vi "Actor Core.vi"(8 "error in":errorcluster, 11 "Display in":refnum<class "Display.lvclass">) -> (0 "error out":errorcluster, 3 "Actor out":refnum<class "Actor.lvclass">)   [LabVIEW 2015, in "UserManagement.lvlib" / "Display.lvclass"]
doc: "(<B>Filename</B>: Actor Framework.lvlib:Actor.lvclass:Actor Core.vi)\n\nReceives messages to the actor, reacts to them, and initiates any error handling that may shut the actor down.\n\nDescendant classes may override this VI to append parallel tasks for the actor to complete while it handles messages. Overrides use the Call Parent Method node."
uses:
  Display.lvclass
  <vilib>/ActorFramework/Actor/Actor.lvclass
  typedef/Main Ctl and UI Ref.ctl
  DatabaseManagement/Database.lvclass
  Display.lvclass/Display.ctl
  userInfoManage/UserInfoManageUI.lvclass
  <vilib>/ActorFramework/Actor/Actor.lvclass/Actor.ctl
  <vilib>/ActorFramework/Message Enqueuer/Message Enqueuer.lvclass/Message Enqueuer.ctl
  Messages/Launch Plugin_Msg/Launch Plugin_Msg.lvclass/Launch Plugin_Msg.ctl
  <vilib>/ActorFramework/Message Enqueuer/Init from Existing Queue.vi
  <vilib>/ActorFramework/Message Enqueuer/Enqueue.vi
  <vilib>/ActorFramework/Message Priority Queue/Priority Enqueue.vi
  <vilib>/ActorFramework/Message Enqueuer/Message Enqueuer.lvclass
  Messages/Launch Plugin_Msg/Launch Plugin_Msg.lvclass
panel:
  out "Info":string
  in  "Tab Control":enum32{"CommonUser", "Admin"}(tab)
  in  "WatchPersonRecord":bool
  in  "Request":bool
  in  "ManageInfo":bool
  in  "WatchEntailInfo":bool
  in  "MakePrintTable":bool
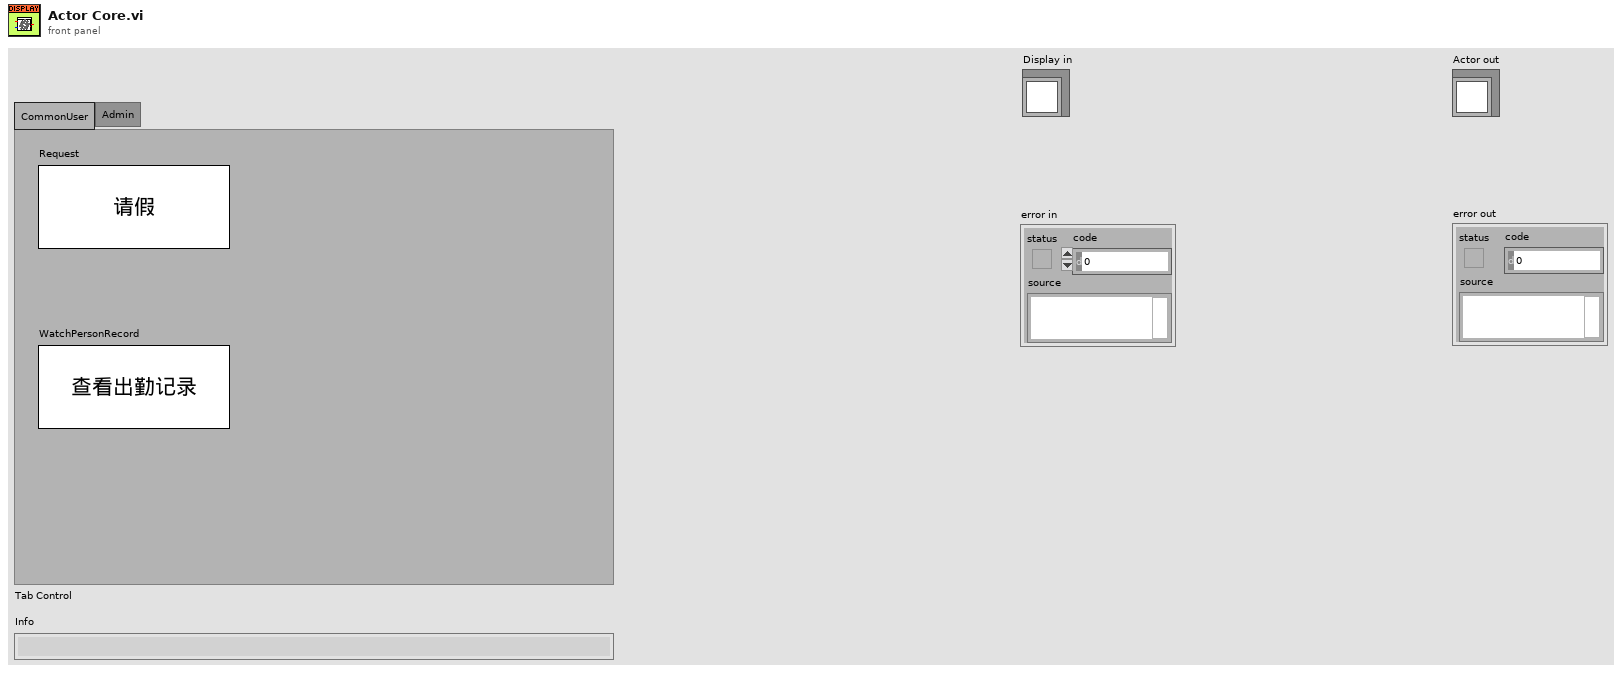
[diagram p1: front panel]
types:
  T1 = typedef "Main Ctl and UI Ref.ctl" = cluster{"Tab Control":refnum<vi>, "Info":refnum<vi>, "This VI":refnum<vi>}
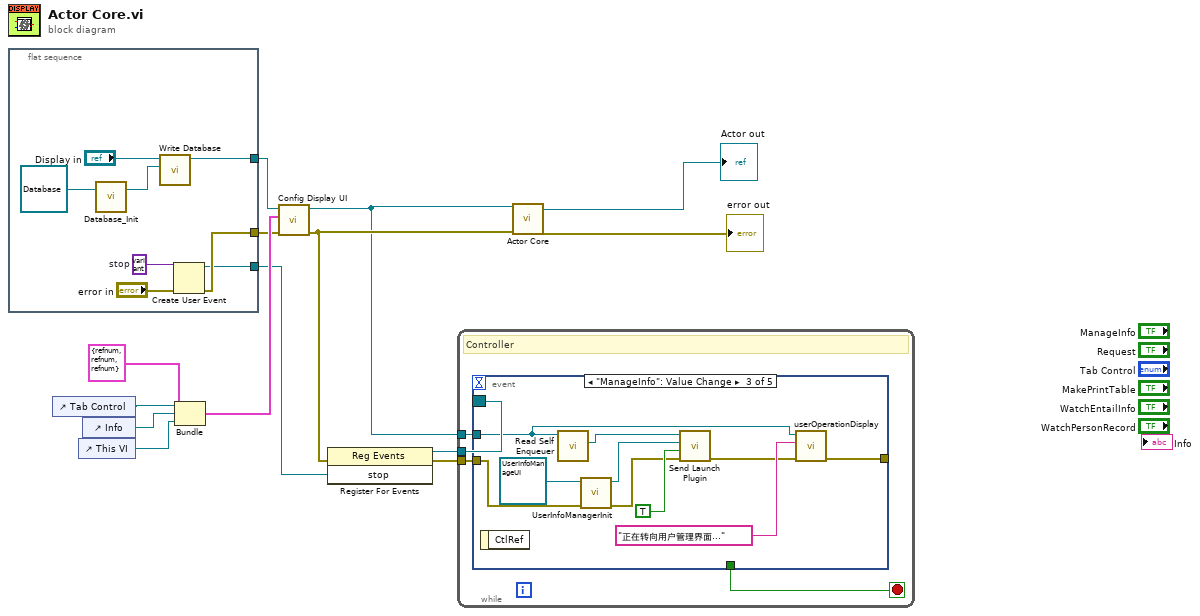
[diagram p0: block diagram]
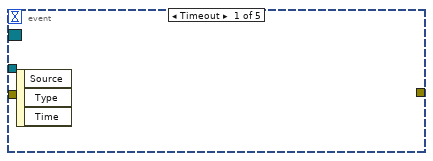
[diagram p2: hidden frame]
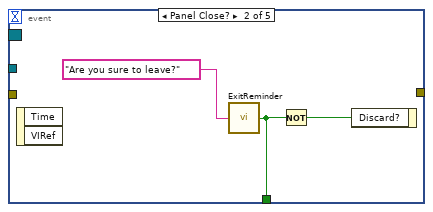
[diagram p3: hidden frame]
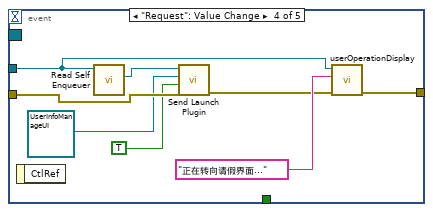
[diagram p4: hidden frame]
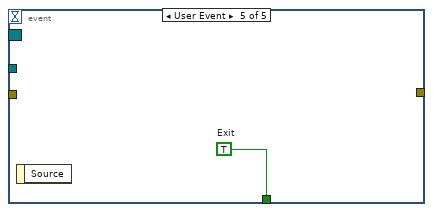
[diagram p5: hidden frame]
diagram:
  n1 = flat-sequence {
    tunnel: [w17] -> w10
    tunnel: [w20] -> w8
    tunnel: [w19] -> w5
    frame #0 {
      w22 = variant  # stop
      n2 = call "Database_Init.vi"("object in"=refnum<class "Database.lvclass"> refnum ("Database.lvlib:Database")) -> ("object out"=w15:refnum<class "Database.lvclass">)  [unwired: 1 in, 1 out]
      n3 = call "Write Database.vi"("Database.lvlib:Database"=w15, "Display in"="Display in") -> ("Display out"=w17:refnum<class "Display.lvclass">)  [unwired: 8 in, 1 out]
      n4 = Create User Event(user event datatype=w22, error in="error in") -> (user event=w19:refnum<user-event>, error out=w20:errorcluster)
    }
  }
  n5 = control-ref of="Tab Control"() -> (w12:refnum<vi>)
  n6 = control-ref of="This VI"() -> (w7:refnum<vi>)
  n7 = control-ref of="Info"() -> (w6:refnum<vi>)
  n8 = Bundle(cluster=T1 {"Tab Control"=refnum, "Info"=refnum, "This VI"=refnum}, "Tab Control"=w12, "Info"=w6, "This VI"=w7) -> (w9:T1)
  n9 = call "Config Display UI.vi"("error in (no error)"=w8, "Main Ctl and UI Ref"=w9, "Management in"=w10) -> ("error out"=w4:errorcluster, "Management out"=w2:refnum<class "Display.lvclass">)  [unwired: 7 in]
  n10 = register-events(error in=w4, w5) -> (reference out=w1:refnum<event-registration>, error out=w3:errorcluster)  [unwired: 1 in]
  n11 = while {
    tunnel: w2 -> [w25]
    tunnel: w3 -> [w24]
    tunnel: w1 -> [w23]
    stop <- w26 stop-if-true
    # "Controller"
    n12 = event shown="[2] \"ManageInfo\": Value Change" {
      selector: w23 -> [_ _ _ _ _]
      dyn-events: _ -> [_ _ _ _ _]
      timeout: _ -> [_ _ _ _ _]
      tunnel: [_ w27 _ _ w48] -> w26
      tunnel: w25 -> [_ _ w36 w43 _]
      tunnel: w24 -> [_ _ w32 w46 _]
      tunnel: [_ _ w35 w42 _] -> _
      event Timeout {
        n13 = event-data() -> ()  [unwired: 1 in, 3 out]
      }
      event Panel Close? {
        n14 = event-data() -> ()  [unwired: 1 in, 2 out]
        n15 = call "ExitReminder.vi"("message"="Are you sure to leave?") -> ("Exit"=w27:bool)
        n16 = Not(x=w27) -> (.not. x?=w28:bool)
        n17 = event-data("Discard?"=w28) -> ()  [unwired: 1 in, 1 out]
      }
      event "ManageInfo": Value Change {
        n18 = event-data() -> ()  [unwired: 1 in, 1 out]
        n19 = call <vilib>:"Read Self Enqueuer.vi"("Actor"=w36) -> ("Self Enqueuer"=w38:refnum<class "Message Enqueuer.lvclass">)  [unwired: 10 in]
        n20 = call "UserInfoManagerInit.vi"("error in (no error)"=w32, "userInfoManage in"=refnum<class "UserInfoManageUI.lvclass"> refnum ("ActorManagement.lvlib:userInfoManage")) -> ("error out"=w30:errorcluster, "userInfoManage out"=w31:refnum<class "UserInfoManageUI.lvclass">)  [unwired: 8 in]
        n21 = call "Send Launch Plugin.vi"("error in (no error)"=w30, "Open Actor Core front panel? (F)"=TRUE, "Plugin.lvclass"=w31, "Message Enqueuer"=w38) -> ("error out"=w37:errorcluster)  [unwired: 6 in, 1 out]
        n22 = call "userOperationDisplay.vi"("error in (no error)"=w37, "Current User Operation"="正在转向用户管理界面...", "Management in"=w36) -> ("error out"=w35:errorcluster)  [unwired: 7 in, 1 out]
      }
      event "Request": Value Change {
        n23 = event-data() -> ()  [unwired: 1 in, 1 out]
        n24 = call <vilib>:"Read Self Enqueuer.vi"("Actor"=w43) -> ("Self Enqueuer"=w45:refnum<class "Message Enqueuer.lvclass">)  [unwired: 10 in]
        n25 = call "Send Launch Plugin.vi"("error in (no error)"=w46, "Open Actor Core front panel? (F)"=TRUE, "Plugin.lvclass"=refnum<class "UserInfoManageUI.lvclass"> refnum ("ActorManagement.lvlib:userInfoManage"), "Message Enqueuer"=w45) -> ("error out"=w44:errorcluster)  [unwired: 6 in, 1 out]
        n26 = call "userOperationDisplay.vi"("error in (no error)"=w44, "Current User Operation"="正在转向请假界面...", "Management in"=w43) -> ("error out"=w42:errorcluster)  [unwired: 7 in, 1 out]
      }
      event User Event {
        w48 = TRUE  # Exit
        n27 = event-data() -> ()  [unwired: 1 in, 1 out]
      }
    }
  }
  n28 = call-parent "Actor Core.vi"("error in"=w4, "Actor in"=w2) -> ("error out"=→"error out":errorcluster, "Actor out"=→"Actor out":refnum<class "Actor.lvclass">)  [unwired: 8 in]
